vi "UpdateMultipleChannels.vi"(8 "error in (no error)":errorcluster, 10 "ChannelsIn":refnum<class "T560Channel.lvclass">[](array[class]), 11 "T560Session in":refnum<class "T560Session.lvclass">) -> (0 "error out":errorcluster, 3 "T560Session out":refnum<class "T560Session.lvclass">)   [LabVIEW 2013, in "T560Session.lvclass"]
doc: "Update multiple channels objects within the current Session object\nIf a specific channel object is not found, it will be added to the Session object"
uses:
  T560Session.lvclass
  T560ChannelClass/T560Channel.lvclass
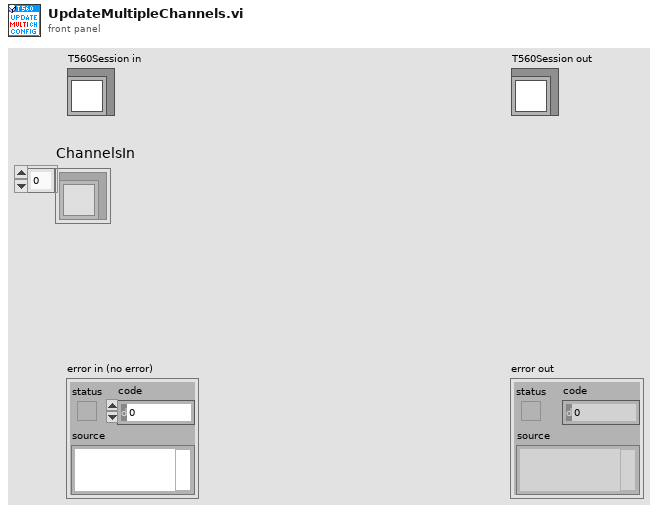
[diagram p1: front panel]
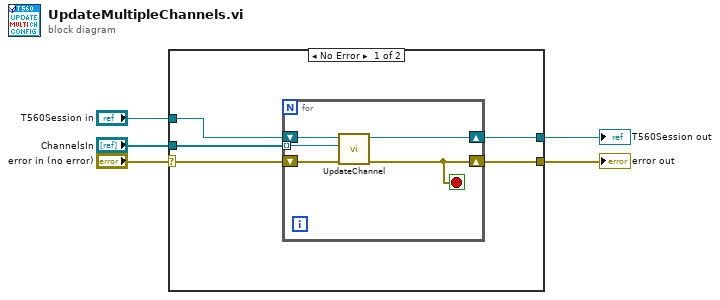
[diagram p0: block diagram]
diagram:
  n1 = case shown="No Error" "error in (no error)" {
    selector: "error in (no error)" -> [w7 w17]
    tunnel: [w6 w17] -> w4
    tunnel: [w8 w16] -> w2
    tunnel: "T560Session in" -> [w10 w16]
    tunnel: "ChannelsIn" -> [w9 _]
    frame No Error {
      n2 = for {
        tunnel: w9 -> [w14] mode=indexing
        shift-right: [w11] -> w6
        shift-left: w7 -> [w12]
        shift-right: [w13] -> w8
        shift-left: w10 -> [w15]
        stop <- w11 stop-if-true
        n3 = call-dynamic "UpdateChannel.vi"("error in"=w12, "UpdatedChannel.lvclass"=w14, "T560Session in"=w15) -> ("error out"=w11:errorcluster, "T560Session out"=w13:refnum<class "T560Session.lvclass">)  [unwired: 7 in]
      }
    }
    frame Error {
    }
  }
  "error out" <- w4
  "T560Session out" <- w2
